vi "Not A Message.vi"(8 "error in (no error)":errorcluster, 11 "Abstract Request Message in":refnum<class "Abstract Request Message.lvclass">) -> (0 "error out":errorcluster, 2 "Not a Message?":bool, 3 "Abstract Request Message out":refnum<class "Abstract Request Message.lvclass">)   [LabVIEW 2017, in "Messaging.lvlib" / "Abstract Request Message.lvclass"]
uses:
  Abstract Request Message.lvclass
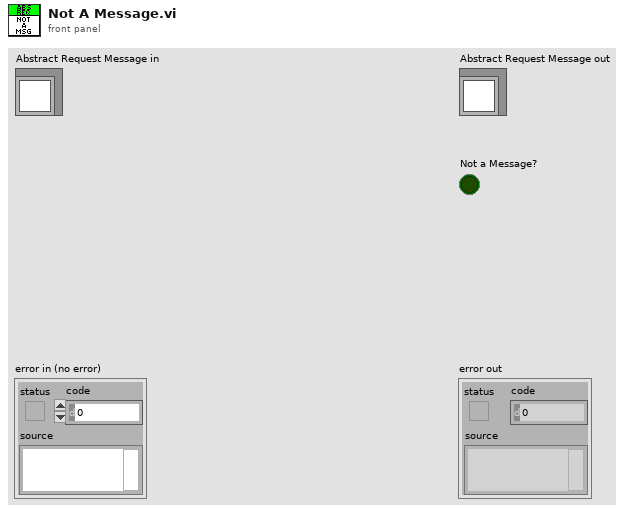
[diagram p1: front panel]
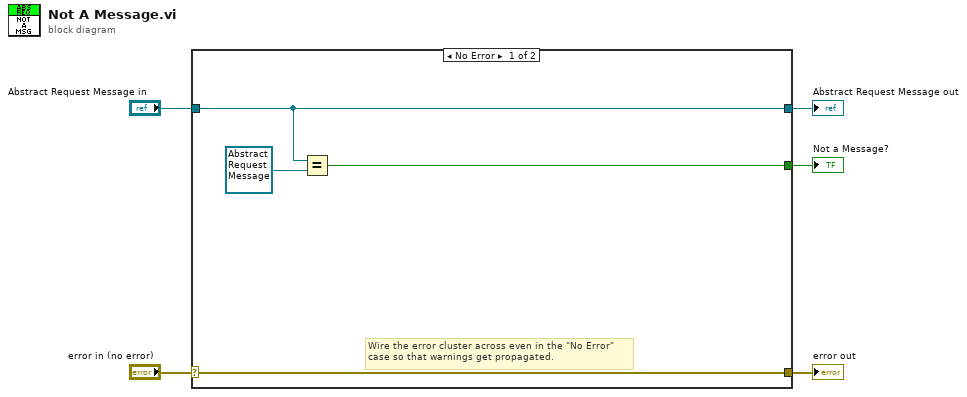
[diagram p0: block diagram]
diagram:
  n1 = case shown="No Error" "error in (no error)" {
    selector: "error in (no error)" -> [w9 w11]
    tunnel: [w9 w11] -> w4
    tunnel: [w7 w10] -> w2
    tunnel: "Abstract Request Message in" -> [w7 w10]
    tunnel: [w6 _] -> w1
    frame No Error {
      # "Wire the error cluster across even in the \"No Error\"\ncase so that warnings get propagated."
      n2 = Equal?(x=w7, y=refnum<class "Abstract Request Message.lvclass"> refnum ("Messaging.lvlib:Message.lvlib:Abstract Request Message.lvclass")) -> (x = y?=w6:bool)
    }
    frame Error {
    }
  }
  "error out" <- w4
  "Abstract Request Message out" <- w2
  "Not a Message?" <- w1
